vi "Ustaw diody kanalow.vi"(4 "LeftD (57)":i32=57, 6 "Left0 (20)":i32=20, 7 "Top (90)":i32=90, 8 "error in (no error)":errorcluster, 10 "AI aktywne array in":refnum<vi>[](array[refnum])) -> (0 "error out":errorcluster)   [LabVIEW 2014]
doc: "Ustawia diody wskazujące aktywność kanałów\nw zakładce Konfiguracja"
uses:
  <vilib>/Utility/miscctls.llb/LVPositionTypeDef.ctl
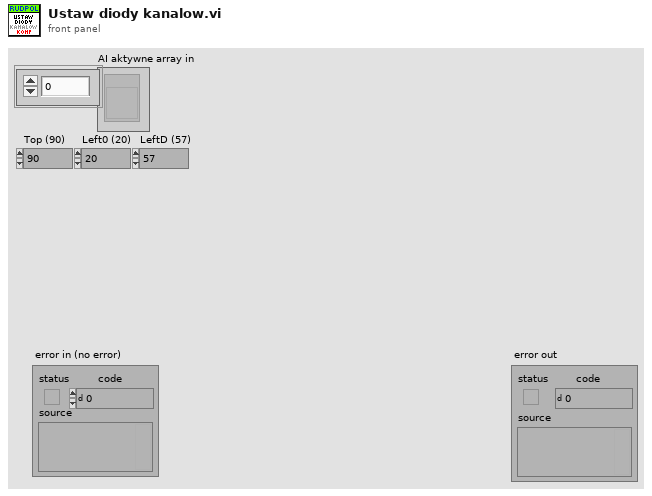
[diagram p1: front panel]
types:
  T1 = typedef "LVPositionTypeDef.ctl" = cluster{"Left":i32, "Top":i32}
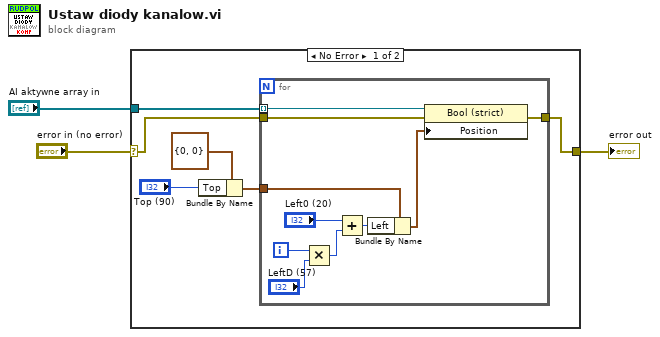
[diagram p0: block diagram]
diagram:
  n1 = case shown="No Error" "error in (no error)" {
    selector: "error in (no error)" -> [w5 w20]
    tunnel: [w4 w20] -> w2
    tunnel: "AI aktywne array in" -> [w9 _]
    frame No Error {
      n2 = Bundle By Name(cluster=T1 {"Left"=0, "Top"=0} ("Position"), "Top"="Top (90)") -> (w6:T1)
      n3 = for {
        tunnel: w9 -> [w19] mode=indexing
        tunnel: w6 -> [w18]
        tunnel: w5 -> [w14]
        tunnel: [w13] -> w4
        i -> [w12]
        n4 = Multiply(x=w12, y="LeftD (57)") -> (x*y=w11:i32)
        n5 = Add(x="Left0 (20)", y=w11) -> (x+y=w15:i32)
        n6 = Bundle By Name(cluster=w18, "Left"=w15) -> (w17:T1)
        n7 = property class="Bool (strict)"(reference=w19, error in=w14, "Position"=w17) -> (error out=w13:errorcluster)  [unwired: 1 out]
      }
    }
    frame Error {
    }
  }
  "error out" <- w2
